vi "PathPlanner_RamseteCtrl_Execute.vi"(4 "Enabled":bool=TRUE, 6 "Reset":bool, 7 "RAMSETE_EXE_TUNING SI":T7={"B"=2.0, "Zeta"=0.7, "X Tolerance M"=2.0, "Y Tolerance M"=0.7, "Heading Tolerance RAD"=0.7, "Track Width M"=2.0, "Max Speed M/S"=2.0} {"Max Speed M/S" format="%13.4f"; "Track Width M" format="%13.4f"; "Heading Tolerance RAD" format="%13.4f"; "Y Tolerance M" format="%13.4f"; "X Tolerance M" format="%13.4f"; "Zeta" format="%13.4f"; "B" format="%13.4f"}, 9 "Current Pose SI":T2={"TRANSLATION"={"X"=0.0, "Y"=0.0}, "ROTATION"={"VALUE"=0.0, "COS"=1.0, "SIN"=0.0}} {"ROTATION"."SIN" format="%13.4f"; "ROTATION"."COS" format="%13.4f"; "ROTATION"."VALUE" format="%13.4f"; "TRANSLATION"."Y" format="%14.3f"; "TRANSLATION"."X" format="%14.3f"}, 11 "PathPlannerState":T5={"TimeSeconds"=0.0, "VelocityMPS"=0.0, "AccerationMpsSq"=0.0, "HeadingAngularVelRadPerSec"=0.0, "PositionMeters"={"X"=0.0, "Y"=0.0}, "Heading"={"VALUE"=0.0, "COS"=1.0, "SIN"=0.0}, "TargetHolonomicRotation"={"VALUE"=0.0, "COS"=1.0, "SIN"=0.0}, "CurvatureRadPerMeter"=0.0, "PathPlannerConstraints"={"MaxVelocityMps;"=0.0, "MaxAccelerationMpsSq;"=0.0, "MaxAngularVelRadPsEc;"=0.0, "MaxAngularAccRadPSecSq"=0.0, "Exists"=FALSE}, "DeltaPos"=0.0} {"TargetHolonomicRotation"."SIN" format="%13.4f"; "TargetHolonomicRotation"."COS" format="%13.4f"; "TargetHolonomicRotation"."VALUE" format="%13.4f"; "Heading"."SIN" format="%13.4f"; "Heading"."COS" format="%13.4f"; "Heading"."VALUE" format="%13.4f"; "PositionMeters"."Y" format="%14.3f"; "PositionMeters"."X" format="%14.3f"}) -> (0 "Position Error M":dbl, 1 "At Reference":bool, 2 "Right Speed Dmd M/S":dbl, 3 "Left Speed Dmd M/S":dbl, 5 "outRAMSETE":T1={"B"=2.0, "Zeta"=0.7, "poseTolerance"={"TRANSLATION"={"X"=0.0, "Y"=0.0}, "ROTATION"={"VALUE"=0.0, "COS"=1.0, "SIN"=0.0}}, "poseError"={"TRANSLATION"={"X"=0.0, "Y"=0.0}, "ROTATION"={"VALUE"=0.0, "COS"=1.0, "SIN"=0.0}}, "Enabled"=TRUE} {"poseError"."ROTATION"."SIN" format="%13.4f"; "poseError"."ROTATION"."COS" format="%13.4f"; "poseError"."ROTATION"."VALUE" format="%13.4f"; "poseError"."TRANSLATION"."Y" format="%14.3f"; "poseError"."TRANSLATION"."X" format="%14.3f"; "poseTolerance"."ROTATION"."SIN" format="%13.4f"; "poseTolerance"."ROTATION"."COS" format="%13.4f"; "poseTolerance"."ROTATION"."VALUE" format="%13.4f"; "poseTolerance"."TRANSLATION"."Y" format="%14.3f"; "poseTolerance"."TRANSLATION"."X" format="%14.3f"; "Zeta" format="%12.3f"; "B" format="%12.3f"})   [LabVIEW 2019, in "PathPlanner24.lvlib"]
uses:
  PathPlanner24.lvlib
  <vilib>/Rock Robotics/WPI/ThirdParty/JAS_Junk/TrajLib/TypeDef/RAMSETE_EXE_TUNING.ctl
  <vilib>/Rock Robotics/WPI/ThirdParty/JAS_Junk/TrajLib/TypeDef/POSE2D.ctl
  <vilib>/Rock Robotics/WPI/ThirdParty/JAS_Junk/TrajLib/TypeDef/TRANSLATION2D.ctl
  <vilib>/Rock Robotics/WPI/ThirdParty/JAS_Junk/TrajLib/TypeDef/ROTATION2D.ctl
  TypeDef/PathPlannerTrajectoryState.ctl
  TypeDef/PathPlannerPathConstraints.ctl
  <vilib>/Rock Robotics/WPI/ThirdParty/JAS_Junk/TrajLib/TypeDef/RAMSETE.ctl
  <vilib>/Rock Robotics/WPI/ThirdParty/JAS_Junk/TrajLib/Pose2d_New_TRRO.vi
  <vilib>/Rock Robotics/WPI/ThirdParty/JAS_Junk/TrajLib/Util_CalcDist.vi
  <vilib>/Rock Robotics/SystemInterfaces/NetworkCommunication/NetComm_UsageReport_report.vi
  <vilib>/Rock Robotics/WPI/ThirdParty/JAS_Junk/TrajLib/Rotation2d_CreateAngle.vi
  <vilib>/Rock Robotics/WPI/ThirdParty/JAS_Junk/TrajLib/Translation2d_Create.vi
  <vilib>/Rock Robotics/WPI/ThirdParty/JAS_Junk/TrajLib/Globals/Util_LibraryGlobals.vi
  <vilib>/Rock Robotics/WPI/ThirdParty/JAS_Junk/TrajLib/Trajectory_Library.lvlib
panel:
  # "Normalized"
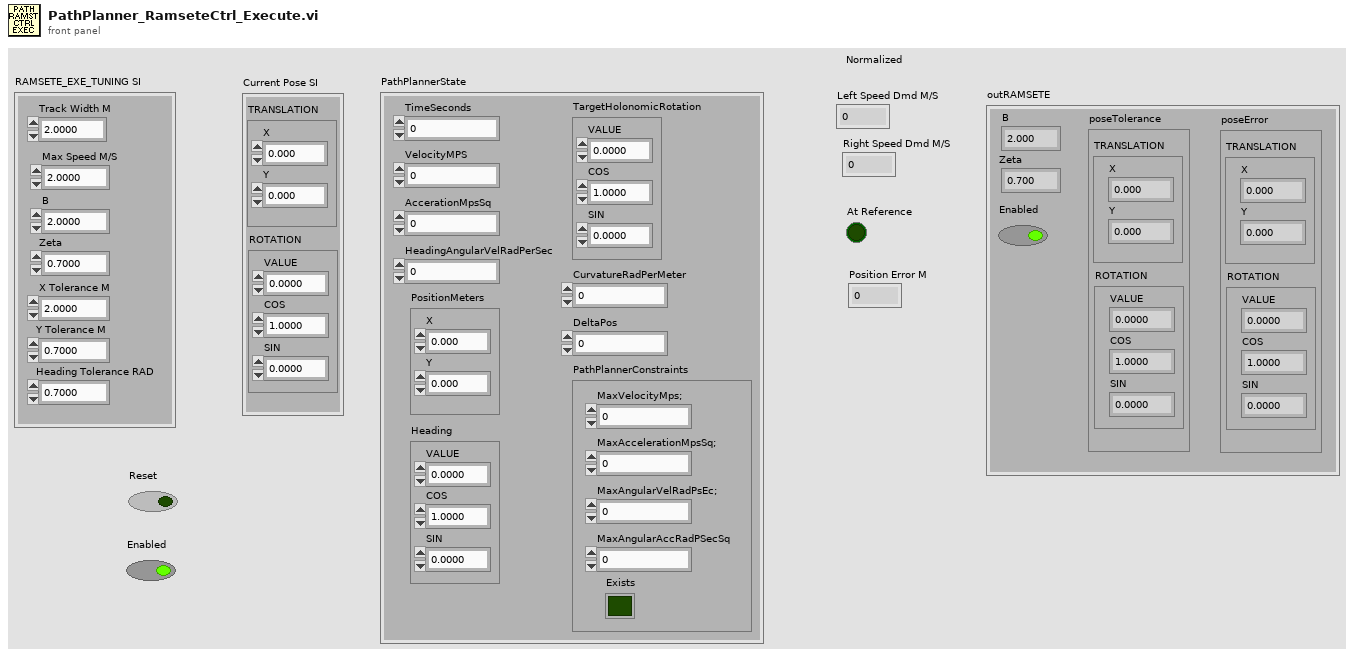
[diagram p1: front panel]
types:
  T1 = typedef "Trajectory_Library.lvlib/RAMSETE.ctl" = cluster{"B":dbl, "Zeta":dbl, "poseTolerance":T2, "poseError":T2, "Enabled":bool}
  T2 = typedef "Trajectory_Library.lvlib/POSE2D.ctl" = cluster{"TRANSLATION":T3, "ROTATION":T4}
  T3 = typedef "Trajectory_Library.lvlib/TRANSLATION2D.ctl" = cluster{"X":dbl, "Y":dbl}
  T4 = typedef "Trajectory_Library.lvlib/ROTATION2D.ctl" = cluster{"VALUE":dbl, "COS":dbl, "SIN":dbl}
  T5 = typedef "PathPlanner24.lvlib/PathPlannerTrajectoryState.ctl" = cluster{"TimeSeconds":dbl, "VelocityMPS":dbl, "AccerationMpsSq":dbl, "HeadingAngularVelRadPerSec":dbl, "PositionMeters":T3, "Heading":T4, "TargetHolonomicRotation":T4, "CurvatureRadPerMeter":dbl, "PathPlannerConstraints":T6, "DeltaPos":dbl}
  T6 = typedef "PathPlanner24.lvlib/PathPlannerPathConstraints.ctl" = cluster{"MaxVelocityMps;":dbl, "MaxAccelerationMpsSq;":dbl, "MaxAngularVelRadPsEc;":dbl, "MaxAngularAccRadPSecSq":dbl, "Exists":bool}
  T7 = typedef "Trajectory_Library.lvlib/RAMSETE_EXE_TUNING.ctl" = cluster{"B":dbl, "Zeta":dbl, "X Tolerance M":dbl, "Y Tolerance M":dbl, "Heading Tolerance RAD":dbl, "Track Width M":dbl, "Max Speed M/S":dbl}
  T8 = typedef "Trajectory_Library.lvlib/DIFF_DRIVE_KINEMATICS.ctl" = cluster{"TrackWidth_Meters":dbl}
  T9 = typedef "Trajectory_Library.lvlib/CHASSIS_SPEEDS.ctl" = cluster{"vX":dbl, "vY":dbl, "vOmega":dbl}
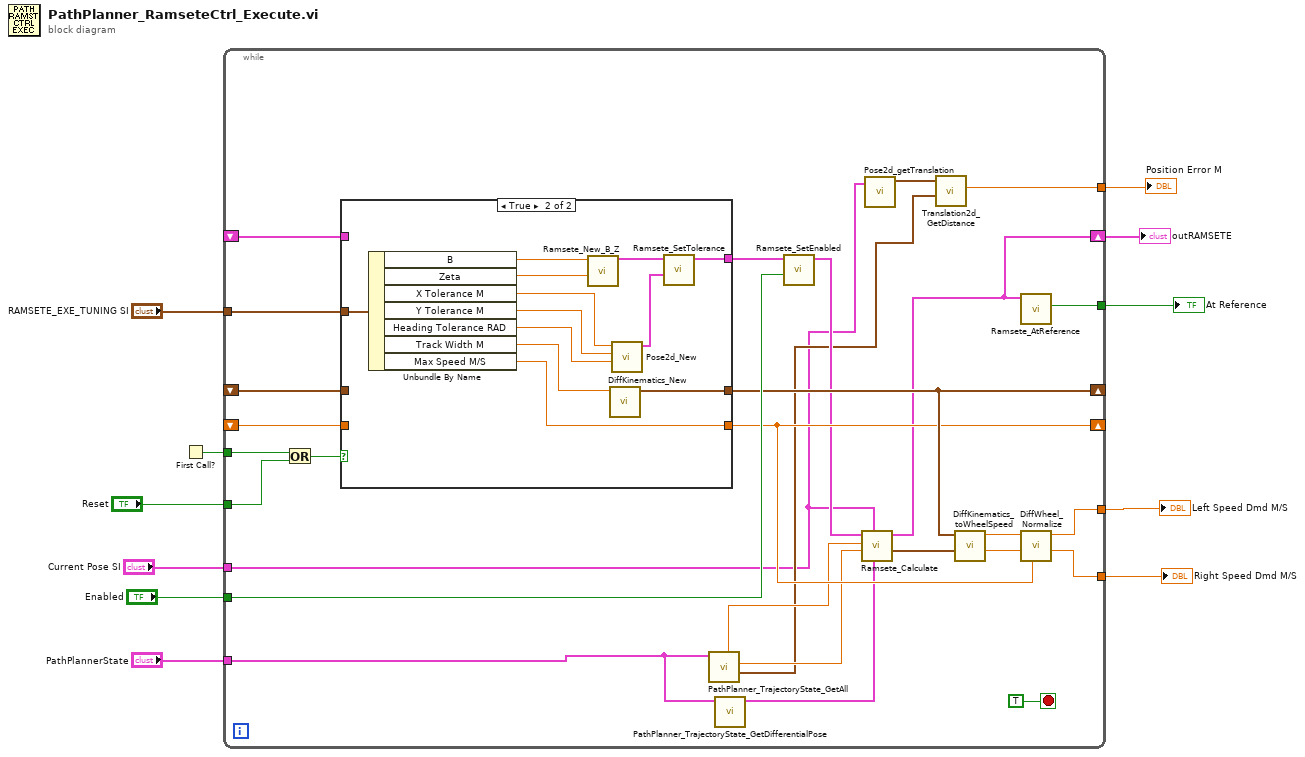
[diagram p0: block diagram]
diagram:
  n1 = First Call?() -> (First Call?: T/F=w10:bool)
  n2 = while {
    tunnel: "RAMSETE_EXE_TUNING SI" -> [w25]
    tunnel: [w37] -> w4
    tunnel: [w36] -> w3
    tunnel: "Enabled" -> [w34]
    tunnel: "Reset" -> [w39]
    tunnel: [w30] -> w5
    tunnel: w10 -> [w33]
    shift-right: [w20] -> w11
    shift-left: _ -> [w32]
    tunnel: "Current Pose SI" -> [w13]
    shift-right: [w27] -> _
    shift-left: _ -> [w26]
    shift-right: [w24] -> _
    shift-left: _ -> [w23]
    tunnel: "PathPlannerState" -> [w19]
    tunnel: [w12] -> w1
    stop <- TRUE stop-if-true
    n3 = Or(x=w33, y=w39) -> (x .or. y?=w38:bool)
    n4 = case shown="True" w38 {
      tunnel: [w42 w52] -> w35
      tunnel: w32 -> [w42 _]
      tunnel: [w41 w51] -> w27
      tunnel: w26 -> [w41 _]
      tunnel: [w40 w43] -> w24
      tunnel: w25 -> [_ w50]
      tunnel: w23 -> [w40 _]
      frame False {
      }
      frame True {
        n5 = Unbundle By Name(w50) -> ("B"=w49:dbl, "Zeta"=w48:dbl, "X Tolerance M"=w47:dbl, "Y Tolerance M"=w46:dbl, "Heading Tolerance RAD"=w45:dbl, "Track Width M"=w44:dbl, "Max Speed M/S"=w43:dbl)
        n6 = call <vilib>:"Ramsete_New_B_Z.vi"("Zeta"=w48, "B"=w49) -> ("outRAMSETE"=w54:T1)  [unwired: 9 in]
        n7 = call <vilib>:"DiffKinematics_New.vi"("TrackWidth_Meters"=w44) -> ("DIFF_DRIVE_KINEMATICS"=w51:T8)  [unwired: 10 in]
        n8 = call <vilib>:"Pose2d_New.vi"("Heading"=w45, "Y"=w46, "X"=w47) -> ("out POSe"=w53:T2)  [unwired: 8 in]
        n9 = call <vilib>:"Ramsete_SetTolerance.vi"("tolerancePose"=w53, "inRAMSETE"=w54) -> ("outRAMSETE"=w52:T1)  [unwired: 9 in]
      }
    }
    n10 = call "PathPlanner_TrajectoryState_GetAll.vi"("PathPlannerState"=w19) -> ("PositionMeters"=w14:T3, "HeadingAngularVelRadPerSec"=w16:dbl, "VelocityMPS"=w17:dbl)  [unwired: 1 in, 7 out]
    n11 = call "PathPlanner_TrajectoryState_GetDifferentialPose.vi"("PathPlannerState"=w19) -> ("DifferentialPose"=w18:T2)  [unwired: 10 in]
    n12 = call <vilib>:"Ramsete_SetEnabled.vi"("Enabled"=w34, "inRAMSETE"=w35) -> ("outRAMSETE"=w22:T1)  [unwired: 9 in]
    n13 = call <vilib>:"Ramsete_Calculate.vi"("DesiredPOSE"=w18, "CurrentPOSE"=w13, "DesiredAngularVelocity"=w16, "DesiredLinearVelocity"=w17, "inRAMSETE"=w22) -> ("CHASSIS Speeds"=w21:T9, "outRAMSETE"=w20:T1)  [unwired: 5 in]
    n14 = call <vilib>:"Pose2d_getTranslation.vi"("in POSE"=w13) -> ("outTRANSLATION"=w15:T3)  [unwired: 10 in]
    n15 = call <vilib>:"Translation2d_GetDistance.vi"("other Translation"=w14, "In Translation"=w15) -> ("Distance"=w12:dbl)  [unwired: 9 in]
    n16 = call <vilib>:"DiffKinematics_toWheelSpeed.vi"("CHASSIS Speed"=w21, "DIFF_DRIVE_KINEMATICS"=w27) -> ("RightVelocity"=w28:dbl, "LeftVelocity"=w29:dbl)  [unwired: 8 in]
    n17 = call <vilib>:"Ramsete_AtReference.vi"("RAMSETE"=w20) -> ("AtReference"=w30:bool)  [unwired: 10 in]
    n18 = call <vilib>:"DiffWheel_Normalize.vi"("Max Speed"=w24, "Right Wheel Demand"=w28, "Left Wheel Demand"=w29) -> ("Normalized Right Wheel Demand"=w36:dbl, "Normalized Left Wheel Demand"=w37:dbl)  [unwired: 7 in]
  }
  "Left Speed Dmd M/S" <- w4
  "Right Speed Dmd M/S" <- w3
  "At Reference" <- w5
  "Position Error M" <- w1
  "outRAMSETE" <- w11
